vi "PSAS.vi"() -> ()   [LabVIEW 2013]
uses:
  user32.dll
  <vilib>/Utility/miscctls.llb/LVCursorListTypeDef.ctl
  <vilib>/Utility/file.llb/Read From Spreadsheet File (DBL).vi
  <vilib>/DAQmx/create/channels.llb/DAQmx Create Channel (CI-Count Edges).vi
  <vilib>/Utility/inputDevices.llb/mouseAcquire.vi
  <vilib>/DAQmx/read.llb/DAQmx Read (Counter U32 1Chan 1Samp).vi
panel:
  out "Cursor - Posição Y ->":dbl
  out "FWMH (eV)":dbl
  in  "Simulao":bool
  out "error out 2":errorcluster
  out "Tensão":dbl[](array[numeric])
  out "Boolean":bool
  in  "type (empty)":string[][](array[string])
  out "FIXO":dbl
  out "iteração":dbl
  out "Simul Value":dbl
  out "error out":errorcluster
  in  "OK Button":bool
  out "max index(es)":i32
  out "Counts":u32[](array[numeric])
  out "Voltage":dbl[](array[numeric])
  out "Data to text file":string
  in  "Clock":enum16{"Start", "Running", "Stop"}(ring)
  in  "Tab Control":enum32{"Painel frontal", "Debug"}(tab)
  in  "Tune":bool
  out "Graph":cluster{dbl[], dbl[]}(graph)
  in  "Time step (ms) step(ms)":dbl=1.7 format="%#_13g"
  in  "Save":bool
  in  "Start":bool
  in  "Stop":bool
  in  "Exit":bool
  out "Time (s)":i32
  out "PCI 6230":bool
  in  "Load":bool
  in  "XX Axis":string(combo)
  out "Max. Peak (eV)            ->":dbl
  out "Actual Potencial (V)    ->":dbl format="%.3f"
  out "Max. Peak Count/s      ->":dbl
  out "Display":string
  in  "Upper Voltage (V)":dbl=4.0
  in  "Lower Voltage (V)":dbl
  in  "Radiation":string(combo)
  in  "Pos. Voltage Adjust (10^-4 V)          ->":dbl=5.0 step=0.1
  in  "Neg. Voltage Adjust (10^-4 V)         ->":dbl=-4.0 step=0.1
  in  "OK Button 2":bool
  in  "Acumular":bool
  in  "OK Button 3":bool
  out "Number of Scans        ->":dbl
  out "Cursor - Posição Y ->  2":dbl
  out "Boolean 2":bool
  out "Waveform Chart":dbl(graph)
  out "data":dbl(graph)
  out "Iteracções/s":i32
  in  "Mode":string(combo)="First run"
  out "Contagens":u32
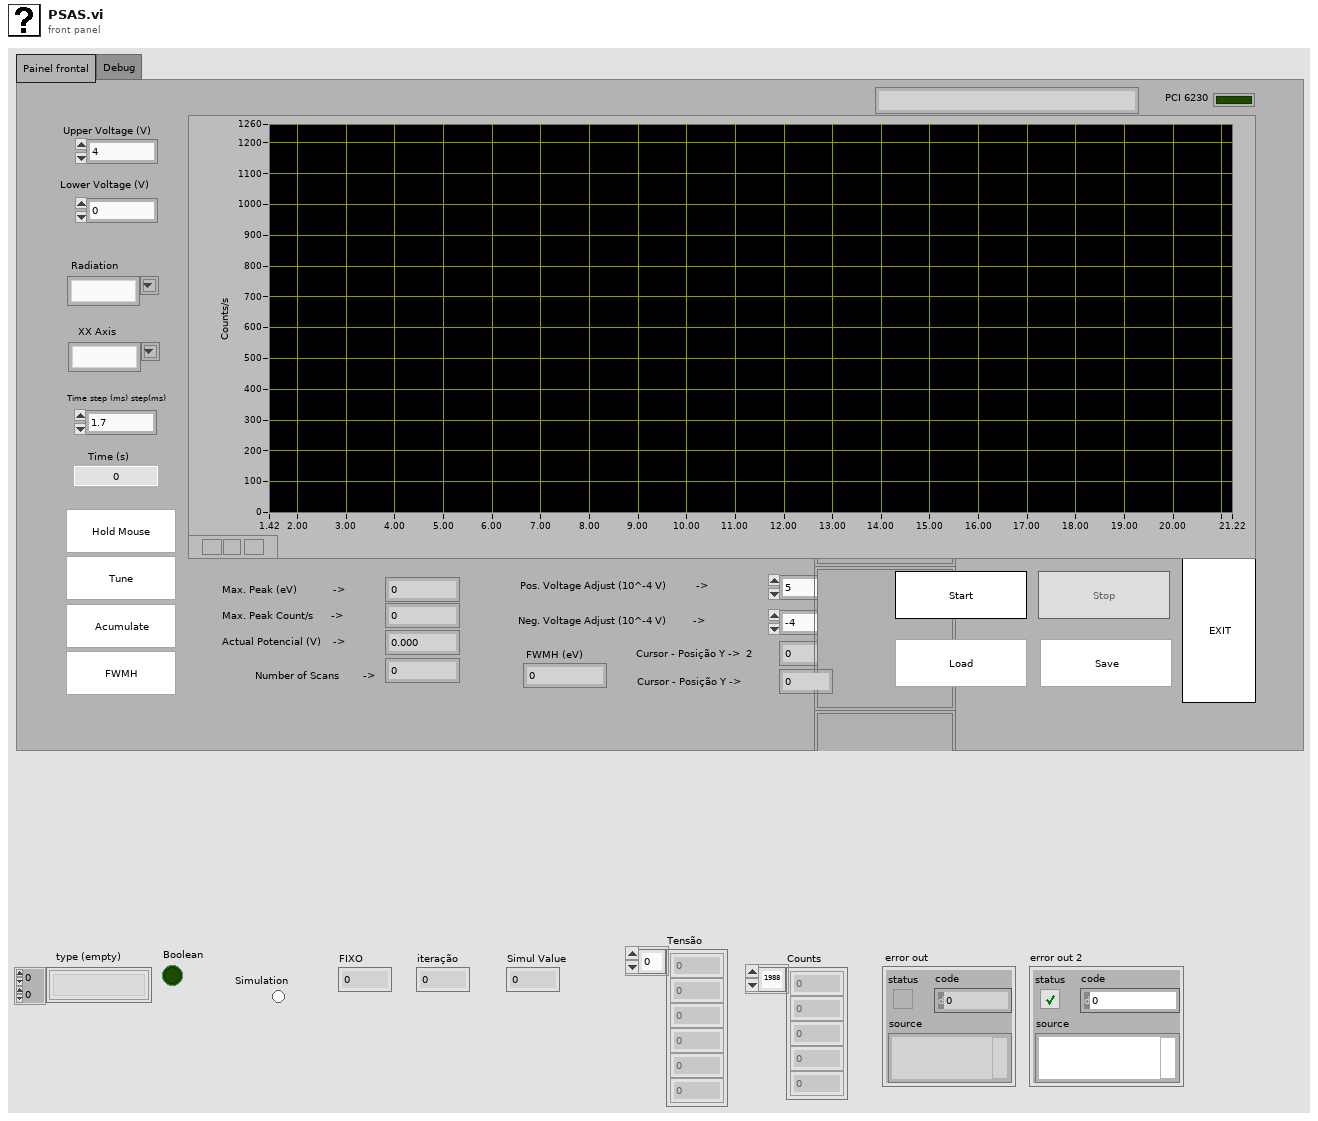
[diagram p1: front panel]
types:
  T1 = typedef "LVCursorListTypeDef.ctl" = cluster{"Name":string, "Color":u32, "Style":u8, "Point Style":u8, "Name Visible":bool, "Allow Drag":bool, "Cursor Mode":u32, "Plot":i32, "Index":i32, "Position":cluster{"X":dbl, "Y":dbl}, "X Scale":u32, "Y Scale":u32, "Watch Plots":i32[], "Watch All Plots":bool, "Plot Area":i32, "Label Offset":cluster{"X":dbl, "Y":dbl}}[]
  T2 = cluster{"Name":string, "Color":u32, "Style":u8, "Point Style":u8, "Name Visible":bool, "Allow Drag":bool, "Cursor Mode":u32, "Plot":i32, "Index":i32, "Position":cluster{"X":dbl, "Y":dbl}, "X Scale":u32, "Y Scale":u32, "Watch Plots":i32[], "Watch All Plots":bool, "Plot Area":i32, "Label Offset":cluster{"X":dbl, "Y":dbl}}
  T3 = enum8{"Enabled", "Disabled", "Disabled and Grayed Out"}
  T4 = enum16{"open", "replace", "create", "open or create", "replace or create", "replace or create with confirmation"}
  T5 = typedef "LVRectTypeDef.ctl" = cluster{"Left":i16, "Top":i16, "Right":i16, "Bottom":i16}
  T6 = cluster{"Name":string, "Color":u32, "Style":u8, "Point Style":u8, "Name Visible":bool, "Allow Drag":bool, "Cursor Mode":u32, "Plot":i32, "Index":i32, "Position":cluster{"X":dbl, "Y":dbl}, "X Scale":u32, "Y Scale":u32, "Watch Plots":i32[], "Watch All Plots":bool, "Plot Area":i32, "Label Offset":cluster{"X":dbl, "Y":dbl}}[]
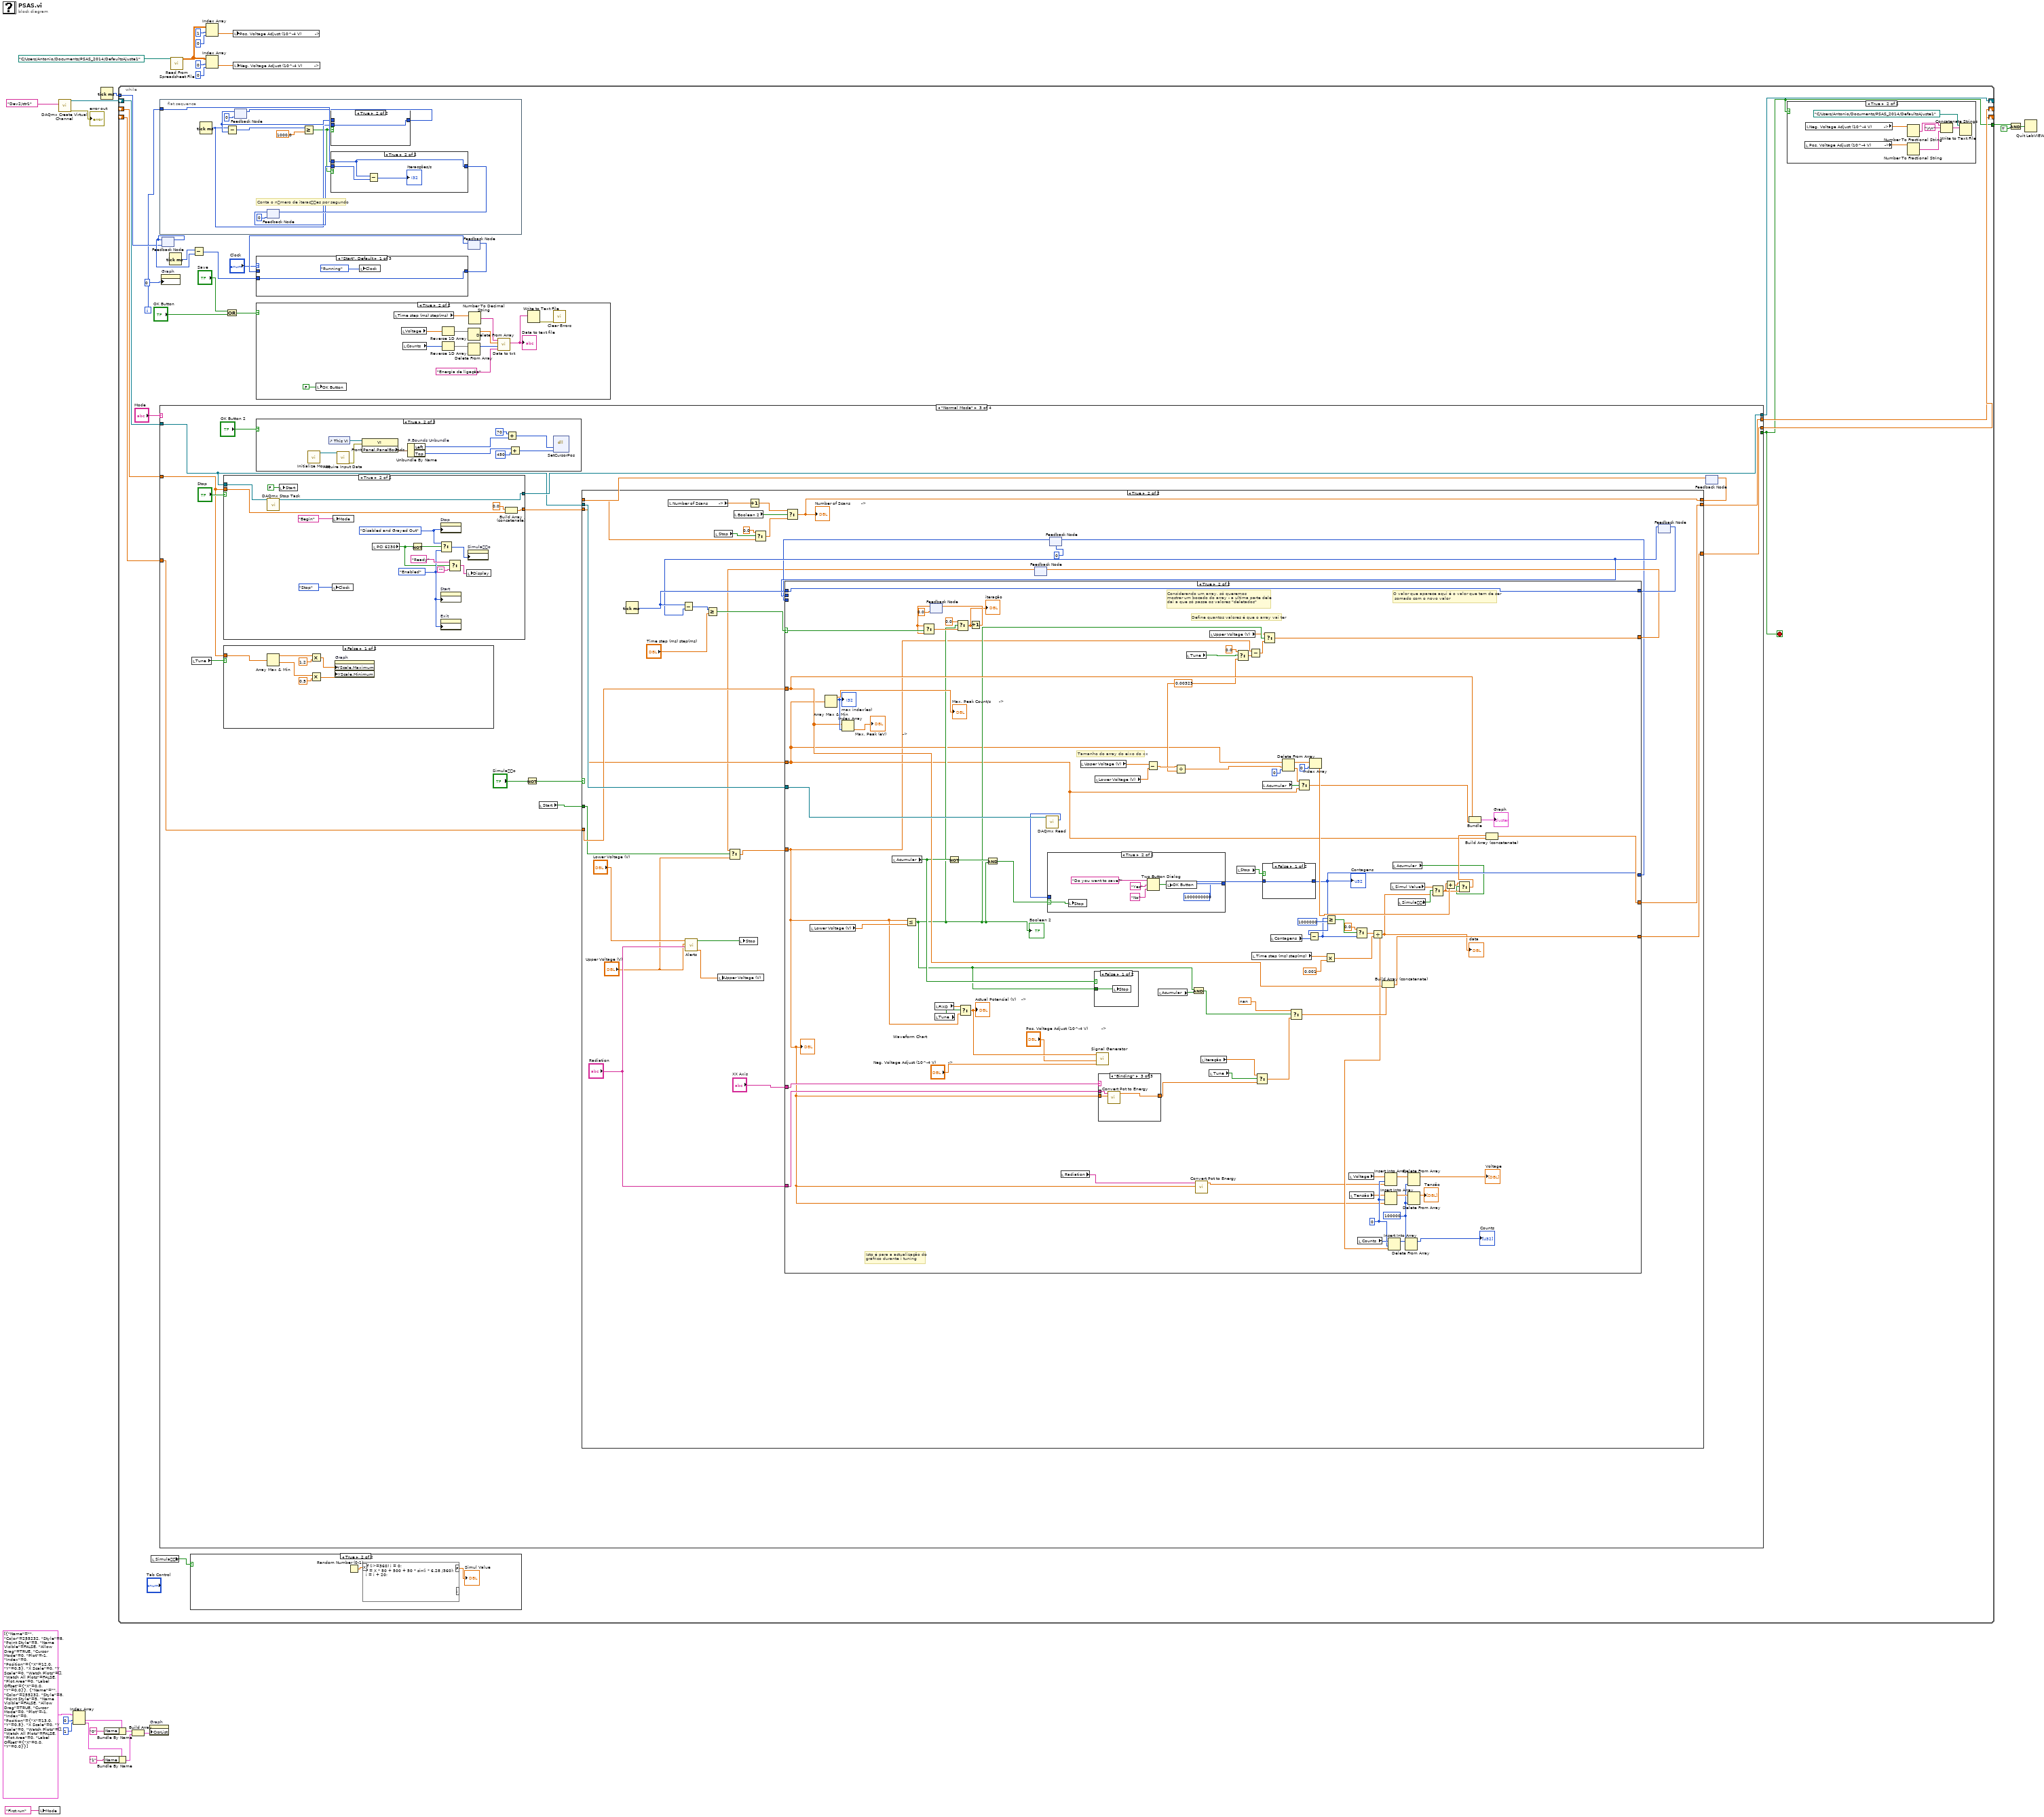
[diagram p0: block diagram]
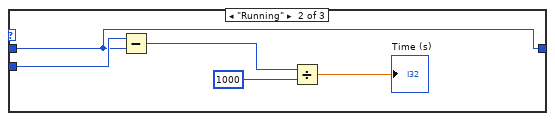
[diagram p5: hidden frame]
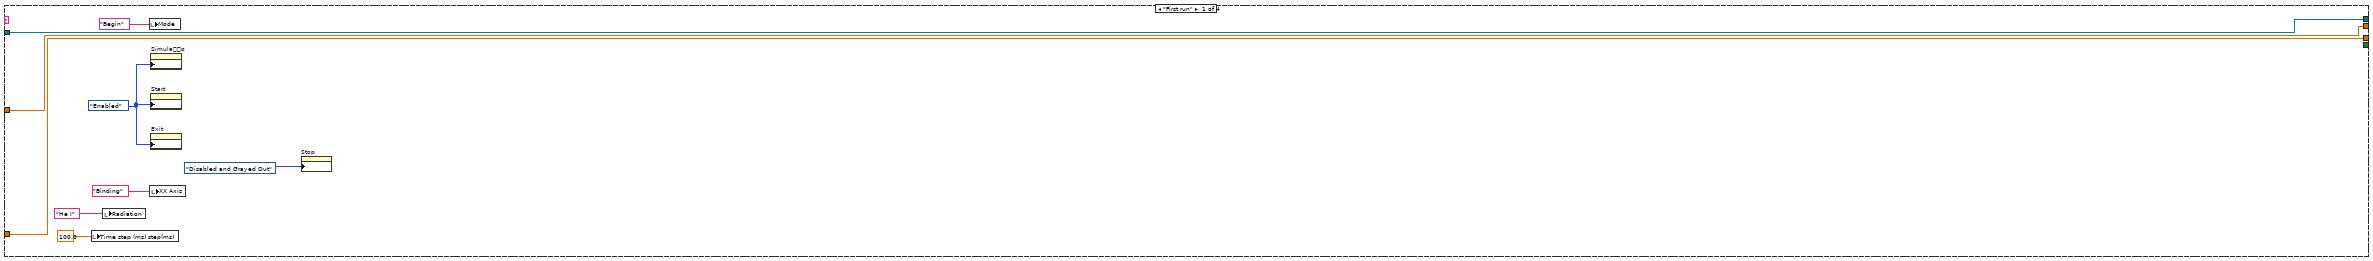
[diagram p9: hidden frame]
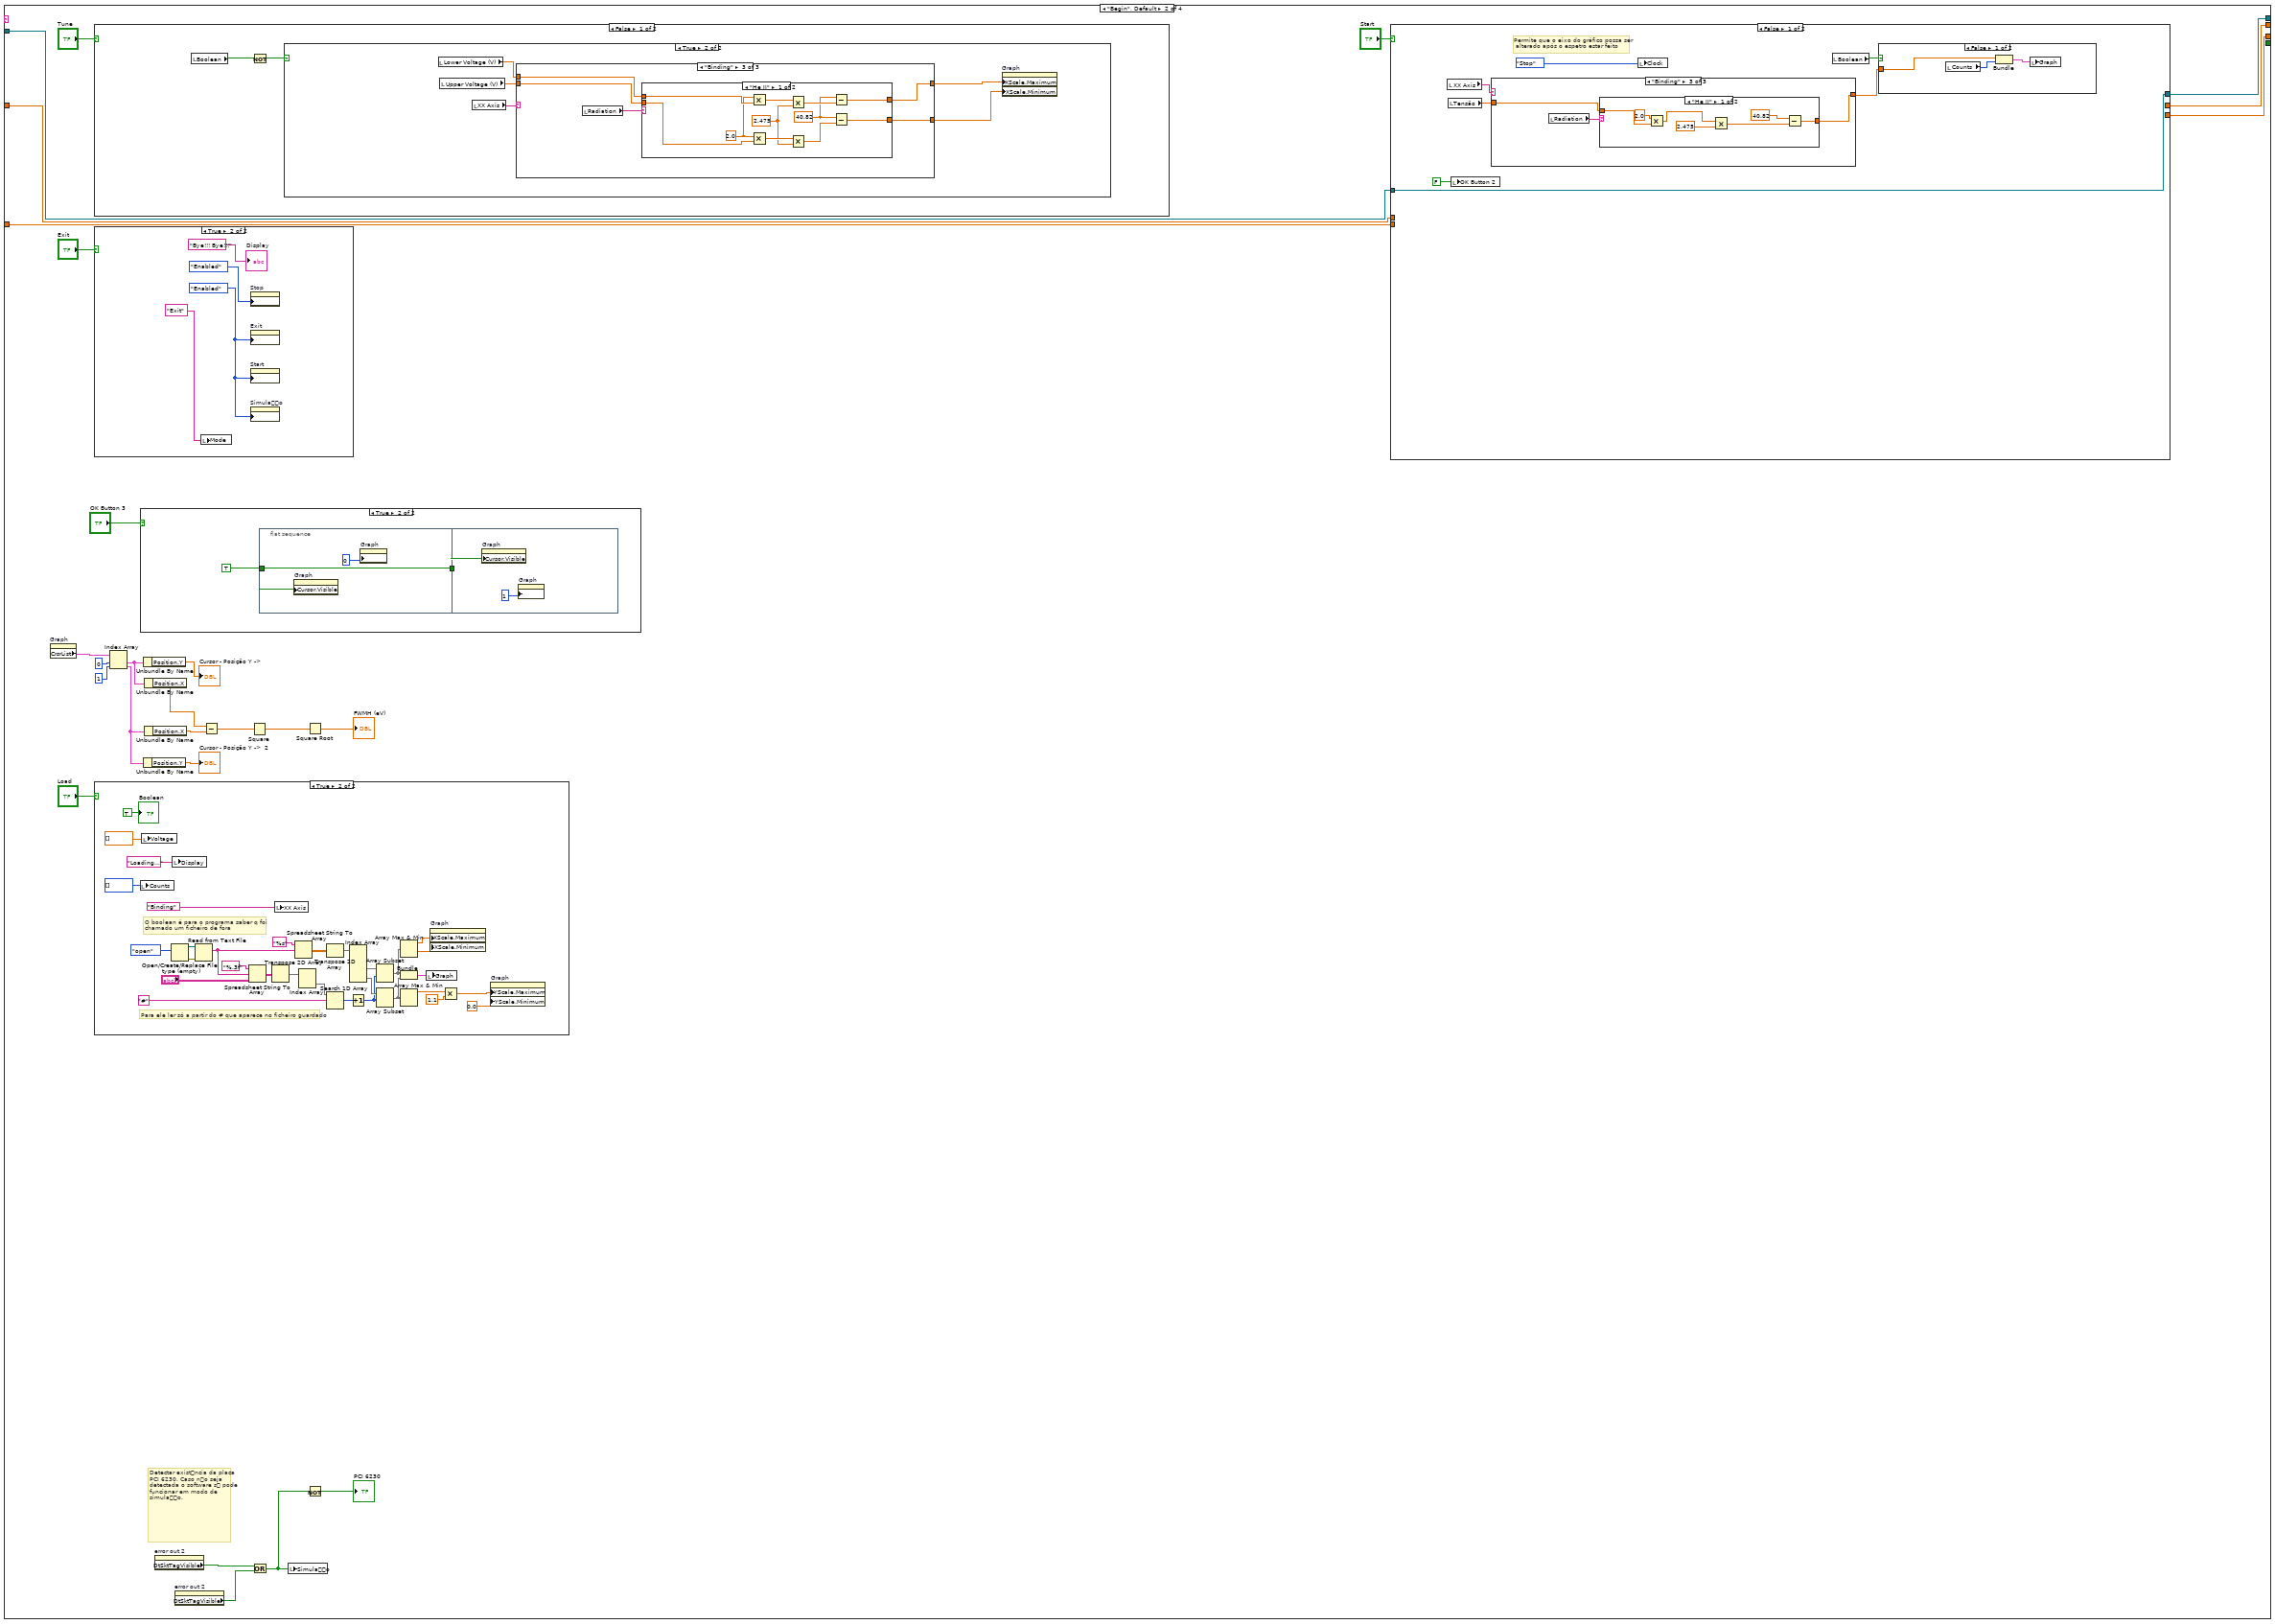
[diagram p10: hidden frame]
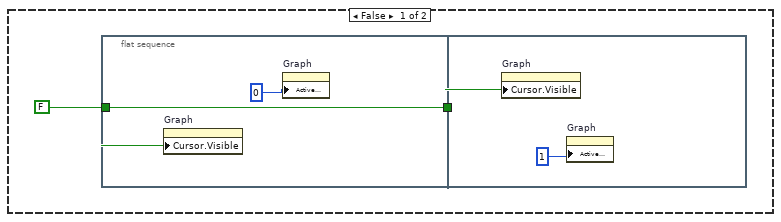
[diagram p11: hidden frame]
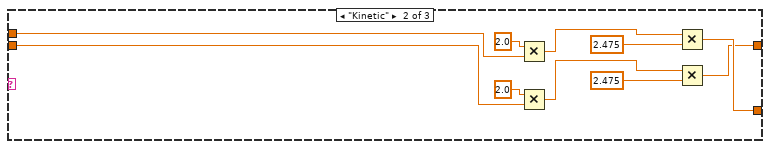
[diagram p14: hidden frame]
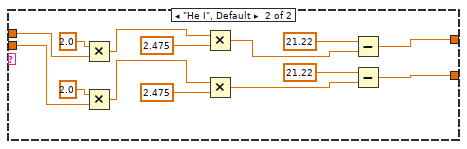
[diagram p15: hidden frame]
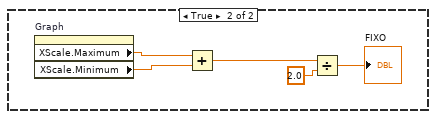
[diagram p16: hidden frame]
diagram:
  n1 = local write "Mode"("First run" ("Mode")) -> ()
  n2 = call-poly <vilib>:"DAQmx Create Virtual Channel.vi"("counter"=tag "Dev2/ctr1") -> ("task out"=w23:refnum<k21>, "error out"=→"error out":errorcluster)  [unwired: 13 in]
  n3 = Index Array(array=T1 [{"Name"="", "Color"=255232, "Style"=8, "Point Style"=5, "Name Visible"=FALSE, "Allow Drag"=TRUE, "Cursor Mode"=0, "Plot"=-1, "Index"=0, "Position"={"X"=12.0, "Y"=0.5}, "X Scale"=0, "Y Scale"=0, "Watch Plots"=[], "Watch All Plots"=FALSE, "Plot Area"=0, "Label Offset"={"X"=0.0, "Y"=0.0}}, {"Name"="", "Color"=255232, "Style"=8, "Point Style"=5, "Name Visible"=FALSE, "Allow Drag"=TRUE, "Cursor Mode"=0, "Plot"=-1, "Index"=0, "Position"={"X"=13.0, "Y"=0.5}, "X Scale"=0, "Y Scale"=0, "Watch Plots"=[], "Watch All Plots"=FALSE, "Plot Area"=0, "Label Offset"={"X"=0.0, "Y"=0.0}}] ("Cursor List"), index #1=0 ("index"), index #2=1 ("index")) -> (element #1=w7:T2, element #2=w4:T2)
  n4 = Tick Count (ms)() -> (millisecond timer value=w26:u32)
  n5 = Bundle By Name(cluster=w7, "Name"="0") -> (w3:T2)
  n6 = Bundle By Name(cluster=w4, "Name"="1") -> (w2:T2)
  n7 = while {
    tunnel: w26 -> [w41]
    shift-right: [w38] -> _
    shift-left: w23 -> [w39]
    shift-right: [w34] -> _
    shift-left: _ -> [w36]
    shift-right: [w33] -> _
    shift-left: _ -> [w35]
    tunnel: [w28] -> w22
    i -> [w37]
    stop <- w28 stop-if-true
    n8 = local read "Simulao"() -> (w29:bool)
    n9 = flat-sequence {
      tunnel: w37 -> [w87]
      frame #0 {
        # "Conta o nmero de iteraces por segundo"
        n10 = Tick Count (ms)() -> (millisecond timer value=w78:u32)
        n11 = feedback #1(u32 0) -> (w80:u32)
        n12 = Subtract(x=w78, y=w80) -> (x-y=w82:u32)
        n13 = feedback #2(0) -> (w85:i32)
        n14 = Greater Or Equal?(x=w82, y=1000.0) -> (x >= y?=w77:bool)
        n15 = case shown="True" w77 {
          tunnel: w78 -> [_ w89]
          tunnel: [w88 w89] -> w81
          tunnel: w80 -> [w88 _]
          frame False {
          }
          frame True {
          }
        }
        n16 = feedback-in #1(w81) -> ()
        n17 = case shown="True" w77 {
          tunnel: w87 -> [_ w91]
          tunnel: [w90 w91] -> w86
          tunnel: w85 -> [w90 w92]
          frame False {
          }
          frame True {
            n18 = Subtract(x=w91, y=w92) -> (x-y=→"Iteracções/s":i32)
          }
        }
        n19 = feedback-in #2(w86) -> ()
      }
    }
    n20 = case shown="\"Normal Mode\"" "Mode" {
      tunnel: [_ _ _ TRUE] -> w28
      tunnel: w39 -> [w100 w128 w291 w504]
      tunnel: [w100 w121 w292 w504] -> w38
      tunnel: [w99 w125 w297 w503] -> w34
      tunnel: w36 -> [w99 w126 w295 w503]
      tunnel: [w98 w124 w296 w502] -> w33
      tunnel: w35 -> [w98 w127 w285 w502]
      frame "First run" {
        w94 = T3."Enabled" ("Disabled")
        n21 = local write "Time step (ms) step(ms)"(100.0 ("Time step(ms)")) -> ()
        n22 = local write "Radiation"("He I" ("Combo Box")) -> ()
        n23 = local write "Mode"("Begin" ("Mode")) -> ()
        n24 = local write "XX Axis"("Binding" ("Combo Box 2")) -> ()
        n25 = property on="Simulao" class="Bool (strict)"("DisabledEnum"=w94) -> ()  [unwired: 2 in, 2 out]
        n26 = property on="Start" class="Bool (strict)"("DisabledEnum"=w94) -> ()  [unwired: 2 in, 2 out]
        n27 = property on="Exit" class="Bool"("DisabledEnum"=w94) -> ()  [unwired: 2 in, 2 out]
        n28 = property on="Stop" class="Bool (strict)"("DisabledEnum"=T3."Disabled and Grayed Out" ("Disabled")) -> ()  [unwired: 2 in, 2 out]
      }
      frame "Begin", Default {
        # "Detectar existncia da placa PCI 6230. Caso no seja detectada o software s pode funcionar em modo de simulao."
        n29 = property on="Graph" class="XYGraph (strict)"() -> ("CrsrList"=w104:T1)  [unwired: 2 in, 2 out]
        n30 = case shown="False" "Tune" {
          frame False {
            n31 = local read "Boolean"() -> (w142:bool)
            n32 = Not(x=w142) -> (.not. x?=w143:bool)
            n33 = case shown="True" w143 {
              frame False {
              }
              frame True {
                n34 = local read "Lower Voltage (V)"() -> (w147:dbl)
                n35 = local read "Upper Voltage (V)"() -> (w145:dbl)
                n36 = local read "XX Axis"() -> (w148:string)
                n37 = case shown="\"Binding\"" w148 {
                  tunnel: [w150 w159 w161] -> w146
                  tunnel: w147 -> [w150 w156 w165]
                  tunnel: w145 -> [w149 w152 w164]
                  tunnel: [w149 w151 w162] -> w144
                  frame "Voltage", Default {
                  }
                  frame "Kinetic" {
                    n38 = Multiply(x=2.0, y=w156) -> (x*y=w158:dbl)
                    n39 = Multiply(x=2.0, y=w152) -> (x*y=w154:dbl)
                    n40 = Multiply(x=w158, y=2.475) -> (x*y=w159:dbl)
                    n41 = Multiply(x=w154, y=2.475) -> (x*y=w151:dbl)
                  }
                  frame "Binding" {
                    n42 = local read "Radiation"() -> (w163:string)
                    n43 = case shown="\"He II\"" w163 {
                      tunnel: [w175 w187] -> w162
                      tunnel: w165 -> [w173 w184]
                      tunnel: w164 -> [w170 w177]
                      tunnel: [w169 w178] -> w161
                      frame "He II" {
                        w166 = 2.0 ("x")
                        w168 = 40.82 ("x")
                        w167 = 2.475 ("y")
                        n44 = Multiply(x=w166, y=w173) -> (x*y=w174:dbl)
                        n45 = Multiply(x=w166, y=w170) -> (x*y=w172:dbl)
                        n46 = Multiply(x=w174, y=w167) -> (x*y=w176:dbl)
                        n47 = Multiply(x=w172, y=w167) -> (x*y=w171:dbl)
                        n48 = Subtract(x=w168, y=w176) -> (x-y=w175:dbl)
                        n49 = Subtract(x=w168, y=w171) -> (x-y=w169:dbl)
                      }
                      frame "He I", Default {
                        n50 = Multiply(x=2.0, y=w184) -> (x*y=w186:dbl)
                        n51 = Multiply(x=2.0, y=w177) -> (x*y=w182:dbl)
                        n52 = Multiply(x=w186, y=2.475) -> (x*y=w189:dbl)
                        n53 = Multiply(x=w182, y=2.475) -> (x*y=w180:dbl)
                        n54 = Subtract(x=21.22, y=w189) -> (x-y=w187:dbl)
                        n55 = Subtract(x=21.22, y=w180) -> (x-y=w178:dbl)
                      }
                    }
                  }
                }
                n56 = property on="Graph" class="XYGraph (strict)"("XScale.Maximum"=w144, "XScale.Minimum"=w146) -> ()  [unwired: 2 in, 2 out]
              }
            }
          }
          frame True {
            n57 = property on="Graph" class="XYGraph (strict)"() -> ("XScale.Maximum"=w191:dbl, "XScale.Minimum"=w192:dbl)  [unwired: 2 in, 2 out]
            n58 = Add(x=w191, y=w192) -> (x+y=w193:dbl)
            n59 = Divide(x=w193, y=2.0) -> (x/y=→"FIXO":dbl)
          }
        }
        n60 = case shown="True" "Exit" {
          frame False {
          }
          frame True {
            w230 = T3."Enabled" ("Disabled")
            n61 = local write "Mode"("Exit" ("Combo Box")) -> ()
            n62 = property on="Stop" class="Bool (strict)"("DisabledEnum"=T3."Enabled" ("Disabled")) -> ()  [unwired: 2 in, 2 out]
            n63 = property on="Exit" class="Bool"("DisabledEnum"=w230) -> ()  [unwired: 2 in, 2 out]
            n64 = property on="Start" class="Bool (strict)"("DisabledEnum"=w230) -> ()  [unwired: 2 in, 2 out]
            n65 = property on="Simulao" class="Bool (strict)"("DisabledEnum"=w230) -> ()  [unwired: 2 in, 2 out]
            "Display" <- "Bye!!! Bye!!!" ("String")
          }
        }
        n66 = case shown="True" "Load" {
          frame False {
          }
          frame True {
            # "O boolean é para o programa saber q foi \nchamado um ficheiro de fora"
            # "Para ele ler só a partir do # que aparece no ficheiro guardado"
            n67 = local write "Counts"(u32[] [] ("Counts")) -> ()
            n68 = local write "Voltage"(dbl[] [] ("Voltage")) -> ()
            n69 = Open/Create/Replace File(operation (0:open)=T4."open") -> (refnum out=w226:refnum<file>, error out=w223:errorcluster)  [unwired: 5 in, 1 out]
            n70 = local write "Display"("Loading..." ("String")) -> ()
            n71 = Read from Text File(file (use dialog)=w226, error in=w223) -> (text=w205:string)  [unwired: 2 in, 3 out]
            n72 = Spreadsheet String To Array(format string="%.3f" ("delimiter (Tab)"), spreadsheet string=w205, array type (2D Dbl)="type (empty)") -> (array=w204:string[][])  [unwired: 1 in]
            n73 = Transpose 2D Array(2D array=w204) -> (transposed array=w203:string[][])
            n74 = local write "XX Axis"("Binding" ("Eixo XX")) -> ()
            n75 = Spreadsheet String To Array(format string="%s", spreadsheet string=w205) -> (array=w222:dbl[][])  [unwired: 2 in]
            n76 = Index Array(array=w203) -> (element=w202:string[])  [unwired: 2 in]
            n77 = Transpose 2D Array(2D array=w222) -> (transposed array=w221:dbl[][])
            n78 = Search 1D Array(1D array=w202, element="#") -> (index of element=w199:i32)  [unwired: 1 in]
            n79 = Index Array(array=w221) -> (element #2=w220:dbl[], element #3=w219:dbl[])  [unwired: 6 in, 1 out]
            n80 = Increment(x=w199) -> (x+1=w198:i32)
            n81 = Array Subset(array=w220, index=w198) -> (w215:dbl[])  [unwired: 1 in]
            n82 = Array Subset(array=w219, index=w198) -> (w212:dbl[])  [unwired: 1 in]
            n83 = Array Max & Min(array=w215) -> (max value=w214:dbl, min value=w213:dbl)  [unwired: 2 out]
            n84 = Bundle(w215, w212) -> (w218:cluster{dbl[], dbl[]})  [unwired: 1 in]
            n85 = Array Max & Min(array=w212) -> (max value=w211:dbl)  [unwired: 3 out]
            n86 = local write "Graph"(w218) -> ()
            n87 = property on="Graph" class="XYGraph (strict)"("XScale.Maximum"=w214, "XScale.Minimum"=w213) -> ()  [unwired: 2 in, 2 out]
            n88 = Multiply(x=w211, y=1.1) -> (x*y=w209:dbl)
            n89 = property on="Graph" class="XYGraph (strict)"("YScale.Maximum"=w209, "YScale.Minimum"=0.0 ("Y Scale.Range:Minimum")) -> ()  [unwired: 2 in, 2 out]
            "Boolean" <- TRUE ("Boolean")
          }
        }
        n90 = Index Array(array=w104, index #1=0 ("index"), index #2=1 ("index")) -> (element #1=w112:T2, element #2=w114:T2)
        n91 = case shown="True" "OK Button 3" {
          frame False {
            n92 = flat-sequence {
              tunnel: FALSE ("Boolean 3") -> [w132]
              tunnel: [w132] -> w131
              tunnel: w131 -> [w134]
              frame #0 {
                n93 = property on="Graph" class="XYGraph (strict)"("Cursor.Visible"=w132) -> ()  [unwired: 2 in, 2 out]
                n94 = property on="Graph" class="XYGraph (strict)"("Active Cursor"=u32 0) -> ()  [unwired: 2 in, 2 out]
              }
              frame #1 {
                n95 = property on="Graph" class="XYGraph (strict)"("Cursor.Visible"=w134) -> ()  [unwired: 2 in, 2 out]
                n96 = property on="Graph" class="XYGraph (strict)"("Active Cursor"=u32 1) -> ()  [unwired: 2 in, 2 out]
              }
            }
          }
          frame True {
            n97 = flat-sequence {
              tunnel: TRUE ("Boolean 3") -> [w138]
              tunnel: [w138] -> w137
              tunnel: w137 -> [w140]
              frame #0 {
                n98 = property on="Graph" class="XYGraph (strict)"("Cursor.Visible"=w138) -> ()  [unwired: 2 in, 2 out]
                n99 = property on="Graph" class="XYGraph (strict)"("Active Cursor"=u32 0) -> ()  [unwired: 2 in, 2 out]
              }
              frame #1 {
                n100 = property on="Graph" class="XYGraph (strict)"("Cursor.Visible"=w140) -> ()  [unwired: 2 in, 2 out]
                n101 = property on="Graph" class="XYGraph (strict)"("Active Cursor"=u32 1) -> ()  [unwired: 2 in, 2 out]
              }
            }
          }
        }
        n102 = Unbundle By Name(w112) -> ("Position.Y"=→"Cursor - Posição Y ->":dbl)
        n103 = Unbundle By Name(w114) -> ("Position.Y"=→"Cursor - Posição Y ->  2":dbl)
        n104 = Unbundle By Name(w112) -> ("Position.X"=w107:dbl)
        n105 = Unbundle By Name(w114) -> ("Position.X"=w108:dbl)
        n106 = property on="error out 2" class="Clust (strict)"() -> ("DtSktTagVisible"=w118:bool)  [unwired: 2 in, 2 out]
        n107 = property on="error out 2" class="Clust (strict)"() -> ("DtSktTagVisible"=w119:bool)  [unwired: 2 in, 2 out]
        n108 = Subtract(x=w107, y=w108) -> (x-y=w109:dbl)
        n109 = Square(x=w109) -> (x^2=w110:dbl)
        n110 = Or(x=w118, y=w119) -> (x .or. y?=w116:bool)
        n111 = local write "Simulao"(w116) -> ()
        n112 = Square Root(x=w110) -> (sqrt(x)=→"FWMH (eV)":dbl)
        n113 = Not(x=w116) -> (.not. x?=→"PCI 6230":bool)
        n114 = case shown="False" "Start" {
          tunnel: w128 -> [w237 w274]
          tunnel: [w237 w273] -> w121
          tunnel: [_ w272] -> w124
          tunnel: w127 -> [_ _]
          tunnel: w126 -> [_ _]
          tunnel: [_ w271] -> w125
          frame False {
            # "Permite que o eixo do gráfico possa ser\n alterado após o espetro estar feito"
            n115 = local read "XX Axis"() -> (w235:string)
            n116 = local read "Tensão"() -> (w234:dbl[])
            n117 = local write "OK Button 2"(FALSE ("OK Button 2")) -> ()
            n118 = case shown="\"Binding\"" w235 {
              tunnel: [w241 w243 w248] -> w233
              tunnel: w234 -> [w241 w242 w247]
              frame "Voltage", Default {
              }
              frame "Kinetic" {
                n119 = Multiply(x=2.0, y=w242) -> (x*y=w245:dbl[])
                n120 = Multiply(x=w245, y=2.475) -> (x*y=w243:dbl[])
              }
              frame "Binding" {
                n121 = local read "Radiation"() -> (w249:string)
                n122 = case shown="\"He II\"" w249 {
                  tunnel: [w253 w260] -> w248
                  tunnel: w247 -> [w250 w257]
                  frame "He II" {
                    n123 = Multiply(x=2.0, y=w250) -> (x*y=w252:dbl[])
                    n124 = Multiply(x=w252, y=2.475) -> (x*y=w255:dbl[])
                    n125 = Subtract(x=40.82, y=w255) -> (x-y=w253:dbl[])
                  }
                  frame "He I", Default {
                    n126 = Multiply(x=2.0, y=w257) -> (x*y=w259:dbl[])
                    n127 = Multiply(x=w259, y=2.475) -> (x*y=w262:dbl[])
                    n128 = Subtract(x=21.22, y=w262) -> (x-y=w260:dbl[])
                  }
                }
              }
            }
            n129 = local write "Clock"(enum16{"Start", "Running", "Stop"}."Stop" ("Clock")) -> ()
            n130 = local read "Boolean"() -> (w232:bool)
            n131 = case shown="False" w232 {
              tunnel: w233 -> [w239 _]
              frame False {
                n132 = local read "Counts"() -> (w238:u32[])
                n133 = Bundle("Tensão"=w239, "Counts"=w238) -> (w240:cluster{"Tensão":dbl[], "Counts":u32[]})  [unwired: 1 in]
                n134 = local write "Graph"(w240) -> ()
              }
              frame True {
              }
            }
          }
          frame True {
            (unwired) 0.0 ("varrimentos")
            w264 = 0.0 ("iteração")
            w266 = dbl[] [] ("Voltage")
            w283 = T3."Disabled and Grayed Out" ("Disabled")
            n135 = call <vilib>:"DAQmx Start Task.vi"("task/channels in"=w274) -> ("task out"=w273:refnum<k21>, "error out"=→"error out 2":errorcluster)  [unwired: 13 in]
            n136 = local write "Start"(FALSE) -> ()
            n137 = local write "Boolean"(FALSE ("Boolean")) -> ()
            n138 = local write "Contagens"(0.0 ("varrimentos")) -> ()
            n139 = local write "Counts"(w266) -> ()
            n140 = local write "Tensão"(w266) -> ()
            n141 = local write "iteração"(w264) -> ()
            n142 = local write "Voltage"(w266) -> ()
            n143 = local write "Number of Scans        ->"(w264) -> ()
            n144 = local read "Simulao"() -> (w281:bool)
            n145 = local write "Clock"(enum16{"Start", "Running", "Stop"}."Start" ("Clock")) -> ()
            n146 = property on="Stop" class="Bool (strict)"("DisabledEnum"=T3."Enabled" ("Disabled")) -> ()  [unwired: 2 in, 2 out]
            n147 = local write "Mode"("Normal Mode" ("Mode")) -> ()
            n148 = Select(t="Simulation mode" ("String"), s=w281, f="Acquisition mode" ("String")) -> (s? t:f=w280:string)
            n149 = local write "Display"(w280) -> ()
            n150 = property on="Simulao" class="Bool (strict)"("DisabledEnum"=w283) -> ()  [unwired: 2 in, 2 out]
            n151 = property on="Start" class="Bool (strict)"("DisabledEnum"=w283) -> ()  [unwired: 2 in, 2 out]
            n152 = property on="Exit" class="Bool"("DisabledEnum"=w283) -> ()  [unwired: 2 in, 2 out]
            n153 = local read "Lower Voltage (V)"() -> (w270:dbl)
            n154 = Initialize Array(w270) -> (w271:dbl[])  [unwired: 1 in]
            n155 = Initialize Array(0.0 ("element")) -> (w272:dbl[])  [unwired: 1 in]
          }
        }
      }
      frame "Normal Mode" {
        n156 = local read "Tune"() -> (w290:bool)
        n157 = case shown="True" "Stop" {
          tunnel: w291 -> [w485 w491]
          tunnel: [w485 w490] -> w292
          tunnel: w285 -> [w483 w487]
          tunnel: [w483 w486] -> w284
          frame False {
            n158 = local write "Start"(TRUE ("Start")) -> ()
          }
          frame True {
            w493 = T3."Disabled and Grayed Out" ("Disabled")
            w496 = T3."Enabled" ("Disabled")
            n159 = call <vilib>:"DAQmx Stop Task.vi"("task/channels in"=w491) -> ("task out"=w490:refnum<k21>)  [unwired: 13 in, 1 out]
            n160 = local write "Start"(FALSE ("Start")) -> ()
            n161 = local write "Clock"(enum16{"Start", "Running", "Stop"}."Stop" ("Clock")) -> ()
            n162 = local write "Mode"("Begin" ("Mode")) -> ()
            n163 = local read "PCI 6230"() -> (w494:bool)
            n164 = Not(x=w494) -> (.not. x?=w495:bool)
            n165 = Select(t=w493, s=w495, f=w496) -> (s? t:f=w501:T3)
            n166 = property on="Stop" class="Bool (strict)"("DisabledEnum"=w493) -> ()  [unwired: 2 in, 2 out]
            n167 = property on="Start" class="Bool (strict)"("DisabledEnum"=w496) -> ()  [unwired: 2 in, 2 out]
            n168 = property on="Exit" class="Bool"("DisabledEnum"=w496) -> ()  [unwired: 2 in, 2 out]
            n169 = Select(t="Ready" ("String"), s=w494, f="") -> (s? t:f=w500:string)
            n170 = local write "Display"(w500) -> ()
            n171 = property on="Simulao" class="Bool (strict)"("DisabledEnum"=w501) -> ()  [unwired: 2 in, 2 out]
            n172 = Build Array (concatenate)(0.0 ("element"), w487) -> (w486:dbl[])
          }
        }
        n173 = case shown="False" w290 {
          tunnel: w285 -> [w309 w316]
          frame False {
            n174 = Array Max & Min(array=w309) -> (max value=w314:dbl, min value=w312:dbl)  [unwired: 2 out]
            n175 = Multiply(x=w314, y=1.2) -> (x*y=w315:dbl)
            n176 = Multiply(x=w312, y=0.5) -> (x*y=w310:dbl)
            n177 = property on="Graph" class="XYGraph (strict)"("YScale.Maximum"=w315, "YScale.Minimum"=w310) -> ()  [unwired: 2 in, 2 out]
          }
          frame True {
            w324 = 100.0 ("y")
            n178 = Split 1D Array(array=w316, index=50) -> (first subarray=w317:dbl[])  [unwired: 1 out]
            n179 = local read "iteração"() -> (w325:dbl)
            n180 = Add(x=w325, y=w324) -> (x+y=w327:dbl)
            n181 = Subtract(x=w325, y=w324) -> (x-y=w326:dbl)
            n182 = Array Max & Min(array=w317) -> (max value=w318:dbl)  [unwired: 3 out]
            n183 = property on="Graph" class="XYGraph (strict)"("XScale.Maximum"=w327, "XScale.Minimum"=w326) -> ()  [unwired: 2 in, 2 out]
            n184 = Multiply(x=w318, y=2.0) -> (x*y=w323:dbl)
            n185 = Multiply(x=w318, y=0.1) -> (x*y=w321:dbl)
            n186 = property on="Graph" class="XYGraph (strict)"("YScale.Maximum"=w323, "YScale.Minimum"=w321) -> ()  [unwired: 2 in, 2 out]
          }
        }
        n187 = case shown="True" "OK Button 2" {
          frame False {
          }
          frame True {
            n188 = call <vilib>:"Initialize Mouse.vi"() -> ("device ID"=w305:refnum<k1>)  [unwired: 10 in, 1 out]
            n189 = control-ref of="This VI"() -> (w308:refnum<vi>)
            n190 = call-poly <vilib>:"Acquire Input Data.vi"("device ID"=w305) -> ("error out"=w307:errorcluster)  [unwired: 15 in, 3 out]
            n191 = property class="VI"(reference=w308, error in=w307) -> ("Front Panel.PanelBounds"=w306:T5)  [unwired: 2 out]
            n192 = Unbundle By Name "P.Bounds Unbundle"(w306) -> ("Left"=w303:i16, "Top"=w304:i16)
            n193 = Add(x=i16 70, y=w303) -> (x+y=w302:i16)
            n194 = Add(x=w304, y=i16 450) -> (x+y=w301:i16)
            n195 = dll-call lib="User32.dll" fn="SetCursorPos"(w302, w301) -> ()  [unwired: 5 in, 3 out]
          }
        }
        n196 = Not(x="Simulao") -> (.not. x?=w287:bool)
        n197 = local read "Start"() -> (w286:bool)
        n198 = feedback #3() -> (w293:dbl)  [unwired: 1 in]
        n199 = case shown="True" w287 {
          tunnel: w291 -> [_ w366]
          tunnel: [w330 w363] -> w297
          tunnel: w295 -> [w330 w361]
          tunnel: [w329 w362] -> w296
          tunnel: w284 -> [w329 w360]
          tunnel: [w328 w351] -> w294
          tunnel: w293 -> [w328 w346]
          tunnel: w286 -> [_ w340]
          frame False {
            n200 = Tick Count (ms)() -> (millisecond timer value=w332:u32)
            n201 = feedback #4() -> (w333:u32)  [unwired: 1 in]
            n202 = Subtract(x=w332, y=w333) -> (x-y=w334:u32)
            n203 = Greater Or Equal?(x=w334, y=u32 100) -> (x >= y?=w335:bool)
            n204 = case shown="True" w335 {
              tunnel: w332 -> [_ w338]
              tunnel: [w337 w338] -> w331
              tunnel: w333 -> [w337 _]
              frame False {
              }
              frame True {
              }
            }
            n205 = feedback-in #4(w331) -> ()
          }
          frame True {
            n206 = Tick Count (ms)() -> (millisecond timer value=w369:u32)
            n207 = local read "Number of Scans        ->"() -> (w344:dbl)
            n208 = call "Alerts.vi"("Radiation type"="Radiation", "Final voltage"="Upper Voltage (V)", "Inicial voltage"="Lower Voltage (V)") -> ("Final voltage"=w352:dbl, "Stop"=w355:bool)  [unwired: 7 in]
            n209 = local read "Stop"() -> (w347:bool)
            n210 = local write "Upper Voltage (V)"(w352) -> ()
            n211 = local read "Boolean 2"() -> (w350:bool)
            n212 = local write "Stop"(w355) -> ()
            n213 = Increment(x=w344) -> (x+1=w349:dbl)
            n214 = Select(t=0.0 ("f"), s=w347, f=w346) -> (s? t:f=w348:dbl)
            n215 = Select(t=w349, s=w350, f=w348) -> (s? t:f=w351:dbl)
            "Number of Scans        ->" <- w351
            n216 = feedback #5() -> (w342:dbl)  [unwired: 1 in]
            n217 = Select(t=w342, s=w340, f="Upper Voltage (V)") -> (s? t:f=w343:dbl)
            n218 = feedback #6(u32 0 ("data")) -> (w364:u32)
            n219 = feedback #7() -> (w368:u32)  [unwired: 1 in]
            n220 = Subtract(x=w369, y=w368) -> (x-y=w356:u32)
            n221 = Greater Or Equal?(x=w356, y="Time step (ms) step(ms)") -> (x >= y?=w354:bool)
            n222 = case shown="True" w354 {
              selector: w354 -> [_ w439]
              tunnel: w369 -> [_ w445]
              tunnel: [w375 w445] -> w370
              tunnel: w368 -> [w375 _]
              tunnel: w343 -> [w374 w377]
              tunnel: [w374 w464] -> w367
              tunnel: w366 -> [_ w463]
              tunnel: [w373 w425] -> w365
              tunnel: w364 -> [w373 _]
              tunnel: [w372 w453] -> w363
              tunnel: w361 -> [w372 w455]
              tunnel: [w371 w450] -> w362
              tunnel: w360 -> [w371 w389]
              tunnel: "XX Axis" -> [_ w452]
              tunnel: "Radiation" -> [_ w451]
              frame False {
              }
              frame True {
                w393 = 0 ("index")
                w392 = 100000 ("index")
                w413 = 0.00323 ("x")
                # "Define quantos valores é que o array vai ter"
                # "O valor que aparece aqui é o valor que tem de ser\n somado com o novo valor"
                # "Isto é para a actualização do\ngráfrico durante i tuning"
                # "Considerando um array, só queremos \nmostrar um bocado do array - a ultima parte dele\ndai a que só passe os valores \"deletados\""
                # "Tamanho do array do eixo do xx"
                n223 = local read "Lower Voltage (V)"() -> (w387:dbl)
                n224 = Array Max & Min(array=w389) -> (max value=→"Max. Peak Count/s      ->":dbl, max index (indices)=w456:i32)  [unwired: 2 out]
                "max index(es)" <- w456
                n225 = Index Array(array=w455, index=w456) -> (element=→"Max. Peak (eV)            ->":dbl)
                n226 = local read "Acumular"() -> (w419:bool)
                n227 = Less Or Equal?(x=w377, y=w387) -> (x <= y?=w404:bool)
                "Boolean 2" <- w404
                n228 = feedback #8(0.0) -> (w437:dbl)
                n229 = Select(t=w437, s=w439, f=w437) -> (s? t:f=w436:dbl)
                n230 = local read "FIXO"() -> (w409:dbl)
                n231 = local read "Tune"() -> (w408:bool)
                n232 = Not(x=w419) -> (.not. x?=w418:bool)
                n233 = Select(t=0.0, s=w404, f=w436) -> (s? t:f=w434:dbl)
                "iteração" <- w434
                n234 = Select(t=w409, s=w408, f=w377) -> (s? t:f=w407:dbl)
                "Actual Potencial (V)    ->" <- w407
                n235 = Increment(x=w434) -> (x+1=w438:dbl)
                n236 = feedback-in #8(w438) -> ()
                n237 = And(x=w418, y=w404) -> (x .and. y?=w417:bool)
                n238 = call-poly <vilib>:"DAQmx Read.vi"("task/channels in"=w463) -> ("data"=w381:u32)  [unwired: 12 in, 2 out]
                n239 = case shown="True" w417 {
                  selector: w417 -> [_ w468]
                  tunnel: w381 -> [w466 _]
                  tunnel: [w466 u32 1000000000 ("data")] -> w380
                  frame False {
                  }
                  frame True {
                    n240 = local write "Stop"(w468) -> ()
                    n241 = Two Button Dialog(message="Do you want to save?", 1:"No" ("F button name (\"Cancel\")"), 2:"Yes" ("T button name (\"OK\")")) -> (T button?=w469:bool)
                    n242 = local write "OK Button"(w469) -> ()
                  }
                }
                n243 = local read "Radiation"() -> (w378:string)
                n244 = local read "Upper Voltage (V)"() -> (w442:dbl)
                n245 = case shown="False" w419 {
                  tunnel: w404 -> [w465 _]
                  frame False {
                    n246 = local write "Stop"(w465) -> ()
                  }
                  frame True {
                  }
                }
                n247 = local read "Lower Voltage (V)"() -> (w441:dbl)
                n248 = call "Signal Generator.vi"("Ajuste Negativo (10 ^-4)"="Neg. Voltage Adjust (10^-4 V)         ->", "Ajuste Positivo (10 ^-4)"="Pos. Voltage Adjust (10^-4 V)          ->", "data"=w407) -> ()  [unwired: 9 in]
                n249 = case shown="\"Binding\"" w452 {
                  tunnel: w377 -> [w474 w477 w480]
                  tunnel: [w474 w478 w482] -> w410
                  tunnel: w451 -> [_ _ w481]
                  frame "Voltage", Default {
                  }
                  frame "Kinetic" {
                    n250 = Multiply(x=2.0, y=w477) -> (x*y=w476:dbl)
                    n251 = Multiply(x=w476, y=2.475) -> (x*y=w478:dbl)
                  }
                  frame "Binding" {
                    n252 = call "Convert Pot to Energy.vi"("Initial Voltage (V)"=w480, "Radiation"=w481) -> ("Energy"=w482:dbl)  [unwired: 9 in]
                  }
                }
                n253 = Subtract(x=w442, y=w441) -> (x-y=w440:dbl)
                n254 = local read "Acumular"() -> (w405:bool)
                n255 = Divide(x=w440, y=w413) -> (x/y=w433:dbl)
                n256 = local read "Tune"() -> (w416:bool)
                n257 = And(x=w404, y=w405) -> (x .and. y?=w403:bool)
                n258 = call "Convert Pot to Energy.vi"("Initial Voltage (V)"=w377, "Radiation"=w378) -> ("Energy"=w376:dbl)  [unwired: 9 in]
                n259 = local read "iteração"() -> (w411:dbl)
                n260 = local read "Tune"() -> (w412:bool)
                n261 = local read "Upper Voltage (V)"() -> (w386:dbl)
                n262 = Select(t=0.0, s=w416, f=w413) -> (s? t:f=w415:dbl)
                n263 = local read "Stop"() -> (w384:bool)
                n264 = Subtract(x=w377, y=w415) -> (x-y=w424:dbl)
                n265 = local read "Time step (ms) step(ms)"() -> (w397:dbl)
                n266 = Select(t=w411, s=w412, f=w410) -> (s? t:f=w406:dbl)
                n267 = local read "Acumular"() -> (w422:bool)
                n268 = case shown="False" w384 {
                  tunnel: w380 -> [w473 _]
                  tunnel: [w473 _] -> w425
                  frame False {
                  }
                  frame True {
                  }
                }
                "Contagens" <- w425
                n269 = Select(t=w386, s=w404, f=w424) -> (s? t:f=w464:dbl)
                n270 = local read "Contagens"() -> (w462:u32)
                n271 = Delete From Array(array=w389, length=w433, index=0) -> (deleted portion=w420:dbl[], array with subset deleted=w426:dbl[])
                n272 = Select(t=nan, s=w403, f=w406) -> (s? t:f=w401:dbl)
                n273 = Select(t=w420, s=w422, f=w389) -> (s? t:f=w430:dbl[])
                n274 = Subtract(x=w425, y=w462) -> (x-y=w379:u32)
                n275 = Index Array(array=w426, index=0) -> (element=w431:dbl)
                n276 = Multiply(x=w397, y=0.001) -> (x*y=w395:dbl)
                n277 = Greater Or Equal?(x=w379, y=u32 1000000) -> (x >= y?=w383:bool)
                n278 = local read "Voltage"() -> (w457:dbl[])
                n279 = local read "Tensão"() -> (w390:dbl[])
                n280 = Select(t=0.0, s=w383, f=w379) -> (s? t:f=w382:dbl)
                n281 = local read "Counts"() -> (w448:u32[])
                n282 = Divide(x=w382, y=w395) -> (x/y=w398:dbl)
                "data" <- w398
                n283 = Build Array (concatenate)(w401, w455) -> (w453:dbl[])
                n284 = Insert Into Array(array=w457, index=w393, new element=w376) -> (w460:dbl[])
                n285 = Insert Into Array(array=w390, index=w393, new element=w377) -> (w394:dbl[])
                n286 = Insert Into Array(array=w448, index=w393, new element=w398) -> (w459:u32[])
                n287 = local read "Simul Value"() -> (w444:dbl)
                n288 = local read "Acumular"() -> (w421:bool)
                n289 = local read "Simulao"() -> (w446:bool)
                n290 = Delete From Array(array=w459, index=w392) -> (array with subset deleted=→"Counts":u32[])  [unwired: 1 in, 1 out]
                n291 = Delete From Array(array=w460, index=w392) -> (array with subset deleted=→"Voltage":dbl[])  [unwired: 1 in, 1 out]
                n292 = Delete From Array(array=w394, index=w392) -> (array with subset deleted=→"Tensão":dbl[])  [unwired: 1 in, 1 out]
                n293 = Select(t=w444, s=w446, f=w398) -> (s? t:f=w428:dbl)
                n294 = Add(x=w428, y=w431) -> (x+y=w429:dbl)
                n295 = Select(t=w429, s=w421, f=w428) -> (s? t:f=w427:dbl)
                n296 = Bundle(w455, w430) -> (→"Graph":cluster{dbl[], dbl[]})  [unwired: 1 in]
                n297 = Build Array (concatenate)(w427, w389) -> (w450:dbl[])
                "Waveform Chart" <- w377
              }
            }
            n298 = feedback-in #5(w367) -> ()
            n299 = feedback-in #6(w365) -> ()
            n300 = feedback-in #7(w370) -> ()
          }
        }
        n301 = feedback-in #3(w294) -> ()
      }
      frame "Exit" {
        n302 = local write "PCI 6230"(FALSE ("PCI 6230")) -> ()
        n303 = local write "Display"("Ready" ("String")) -> ()
        n304 = local write "Mode"("Begin" ("Mode")) -> ()
      }
    }
    n305 = property on="Graph" class="XYGraph (strict)"("Active Cursor"=u32 0) -> ()  [unwired: 2 in, 2 out]
    n306 = feedback #9(w41) -> (w46:u32)
    n307 = feedback-in #9(w46) -> ()
    n308 = Tick Count (ms)() -> (millisecond timer value=w47:u32)
    n309 = case shown="True" w29 {
      frame False {
      }
      frame True {
        n310 = Random Number (0-1)() -> (number: 0 to 1=w55:dbl)
        n311 = formula code="if (i>=360) i = 0;\nF = X * 50 + 500 + 50 * sin(i * 6.28 /360);\ni = i + 20;"("X"=w55) -> ("F"=→"Simul Value":dbl)  [unwired: 1 out]
      }
    }
    n312 = Subtract(x=w47, y=w46) -> (x-y=w45:u32)
    n313 = Or(x="Save", y="OK Button") -> (x .or. y?=w31:bool)
    n314 = case shown="True" w31 {
      frame False {
      }
      frame True {
        n315 = local write "OK Button"(FALSE ("OK Button")) -> ()
        n316 = local read "Time step (ms) step(ms)"() -> (w59:dbl)
        n317 = local read "Voltage"() -> (w68:dbl[])
        n318 = local read "Counts"() -> (w66:u32[])
        n319 = Reverse 1D Array(array=w68) -> (reversed array=w67:dbl[])
        n320 = Reverse 1D Array(array=w66) -> (reversed array=w65:u32[])
        n321 = Delete From Array(array=w67) -> (array with subset deleted=w64:dbl[])  [unwired: 2 in, 1 out]
        n322 = Delete From Array(array=w65) -> (array with subset deleted=w63:u32[])  [unwired: 2 in, 1 out]
        n323 = Number To Decimal String(number=w59) -> (decimal integer string=w58:string)  [unwired: 1 in]
        n324 = call "Data to txt.vi"("Eixo"="Energia de ligação", "2nd column array"=w63, "1st column array"=w64, "Timestep"=w58) -> ("Data to text file"=w62:string)  [unwired: 7 in]
        "Data to text file" <- w62
        n325 = Write to Text File(text=w62) -> (error out=w61:errorcluster)  [unwired: 3 in, 2 out]
        n326 = call <vilib>:"Clear Errors.vi"("error in (no error)"=w61) -> ()  [unwired: 6 in, 1 out]
      }
    }
    n327 = feedback #10() -> (w43:u32)  [unwired: 1 in]
    n328 = case shown="\"Start\", Default" "Clock" {
      tunnel: w45 -> [w70 w75 _]
      tunnel: [w70 w74 w76] -> w44
      tunnel: w43 -> [_ w74 w76]
      frame "Start", Default {
        n329 = local write "Clock"(enum16{"Start", "Running", "Stop"}."Running" ("Enum")) -> ()
      }
      frame "Running" {
        n330 = Subtract(x=w75, y=w74) -> (x-y=w73:u32)
        n331 = Divide(x=w73, y=u32 1000) -> (x/y=→"Time (s)":dbl)
      }
      frame "Stop" {
      }
    }
    n332 = feedback-in #10(w44) -> ()
    n333 = case shown="True" w28 {
      frame False {
      }
      frame True {
        n334 = local read "Pos. Voltage Adjust (10^-4 V)          ->"() -> (w49:dbl)
        n335 = local read "Neg. Voltage Adjust (10^-4 V)         ->"() -> (w50:dbl)
        n336 = Number To Fractional String(number=w50) -> (F-format string=w53:string)  [unwired: 3 in]
        n337 = Number To Fractional String(number=w49) -> (F-format string=w48:string)  [unwired: 3 in]
        n338 = Concatenate Strings(w53, "\r\n", w48) -> (w52:string)
        n339 = Write to Text File(file (use dialog)=path "C:/Users/Antonio/Documents/PSAS_2014/DefaultsAjuste1", text=w52) -> ()  [unwired: 2 in, 3 out]
      }
    }
  }
  n340 = Build Array(w3, w2) -> (w1:T6)
  n341 = property on="Graph" class="XYGraph (strict)"("CrsrList"=w1) -> ()  [unwired: 2 in, 2 out]
  n342 = call-poly <vilib>:"Read From Spreadsheet File.vi"("file path (dialog if empty)"=path "C:/Users/Antonio/Documents/PSAS_2014/DefaultsAjuste1" ("file (use dialog)")) -> ("all rows"=w15:dbl[][])  [unwired: 6 in, 4 out]
  n343 = Index Array(array=w15, index (row)=1, index (col)=0) -> (element=w12:dbl)
  n344 = Index Array(array=w15, index (row)=0, index (col)=0) -> (element=w11:dbl)
  n345 = local write "Pos. Voltage Adjust (10^-4 V)          ->"(w12) -> ()
  n346 = local write "Neg. Voltage Adjust (10^-4 V)         ->"(w11) -> ()
  n347 = And(x=w22, y=TRUE) -> (x .and. y?=w20:bool)
  n348 = Quit LabVIEW(quit? (T)=w20) -> ()
